vi "Initialize Attributes.vi"(8 "error in (no error)":errorcluster, 10 "Attribute Data":variant, 11 "Beep in":refnum<class "Beep.lvclass">) -> (0 "error out":errorcluster, 2 "Found?":bool, 3 "Beep out":refnum<class "Beep.lvclass">)   [LabVIEW 2016, in "CS++BeepActor.lvlib" / "Beep.lvclass"]
doc: "Initialize object attribute.\n\nUnique resources should be allocated elsewhere!"
uses:
  Beep.lvclass
  C:/User/Brand/LVP/TASCA/UTCS/Packages/CSPP_Core/Actors/CS++BaseActor/CS++BaseActor.lvclass
  CSPP_Core/Actors/CS++BaseActor/CS++BaseActor.lvclass/CS++BaseActor.ctl
  Beep.lvclass/Beep.ctl
  CSPP_Core/Actors/CS++BaseActor/CS++BaseActor.lvclass
  CSPP_Core/Libraries/Utilities/CS++Utilities.lvlib
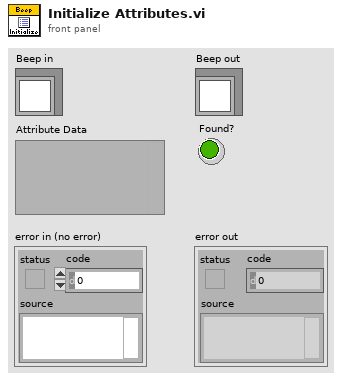
[diagram p1: front panel]
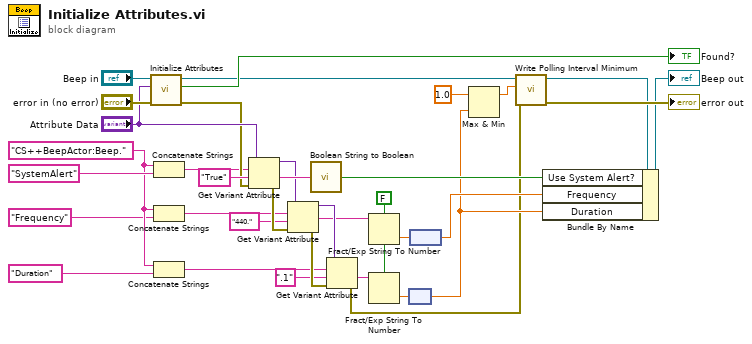
[diagram p0: block diagram]
diagram:
  w6 = FALSE ("use system decimal point (T)")
  w18 = "CS++BeepActor:Beep."
  n1 = call-parent "Initialize Attributes.vi"("error in (no error)"="error in (no error)", "Attribute Data"="Attribute Data", "CS++BaseActor in"="Beep in") -> ("error out"=w28:errorcluster, "Found?"=→"Found?":bool, "CS++BaseActor out"=w31:refnum<class "Beep.lvclass">)  [unwired: 6 in]
  n2 = Concatenate Strings(w18, "SystemAlert") -> (w20:string)
  n3 = Concatenate Strings(w18, "Frequency") -> (w19:string)
  n4 = Concatenate Strings(w18, "Duration") -> (w15:string)
  n5 = Get Variant Attribute(Variant="Attribute Data", name=w20, default value (empty Variant)="True", error in=w28) -> (duplicate Variant=w21:variant, value=w26:string, error out=w22:errorcluster)  [unwired: 1 out]
  n6 = Get Variant Attribute(Variant=w21, name=w19, default value (empty Variant)="440.", error in=w22) -> (duplicate Variant=w16:variant, value=w14:string, error out=w17:errorcluster)  [unwired: 1 out]
  n7 = call "Boolean String to Boolean.vi"("T/F String"=w26) -> ("Value"=w23:bool)
  n8 = Get Variant Attribute(Variant=w16, name=w15, default value (empty Variant)=".1", error in=w17) -> (value=w5:string, error out=w1:errorcluster)  [unwired: 2 out]
  n9 = Fract/Exp String To Number(use system decimal point (T)=w6, string=w14) -> (number=w13:dbl)  [unwired: 2 in, 1 out]
  n10 = Fract/Exp String To Number(use system decimal point (T)=w6, string=w5) -> (number=w7:dbl)  [unwired: 2 in, 1 out]
  n11 = node(w7) -> (w4:dbl[unit])
  n12 = node(w13) -> (w12:dbl[unit])
  n13 = Max & Min(x=dbl[unit] 1.0 ("Polling Interval Minimum"), y=w4) -> (max(x,y)=w2:dbl[unit])  [unwired: 1 out]
  n14 = call "Write Polling Interval Minimum.vi"("error in (no error)"=w1, "Polling Interval Minimum"=w2, "CS++BaseActor in"=w31) -> ("error out"=→"error out":errorcluster, "CS++BaseActor out"=w25:refnum<class "Beep.lvclass">)  [unwired: 7 in]
  n15 = Bundle By Name(cluster=w25, "Use System Alert?"=w23, "Frequency"=w12, "Duration"=w4) -> (→"Beep out":refnum<class "Beep.lvclass">)
